vi "Acquire Data.vi"(4 "amplitude\nsweetspot":dbl, 6 "frequency\nsweetspot":dbl, 7 "error":bool, 10 "Amplitude":dbl, 11 "Frequency":dbl) -> (2 "FFTs":waveform(dbl)[](array[waveform]), 3 "Waveforms":waveform(dbl)[](array[waveform]))   [LabVIEW 2025, in "MCP Demo Application.lvlib"]
uses:
  MCP Demo Application.lvlib
  <vilib>/express/express analysis/Spectral/Block/exnSpectralBlock spectral measurements RMS poly.vi
  <vilib>/express/express analysis/Spectral/Block/exnSpectralBlock spectral measurements RMS array WFM.vi
  <vilib>/express/express analysis/Spectral/XNode/ExpressSpectralMeasurementsBlockNode.xnode
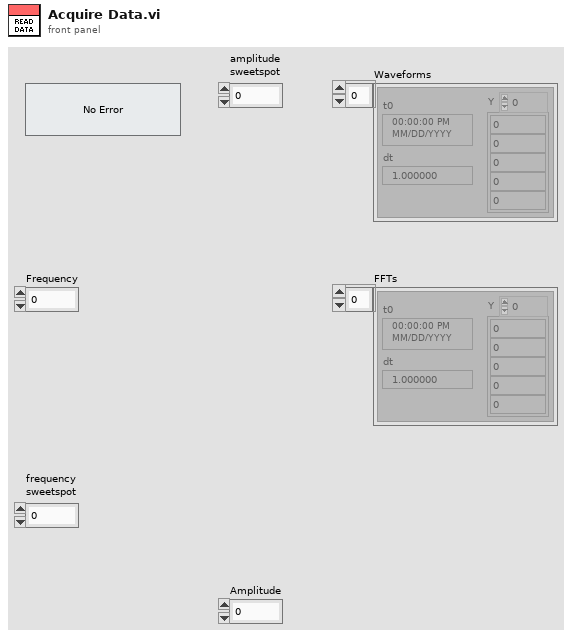
[diagram p1: front panel]
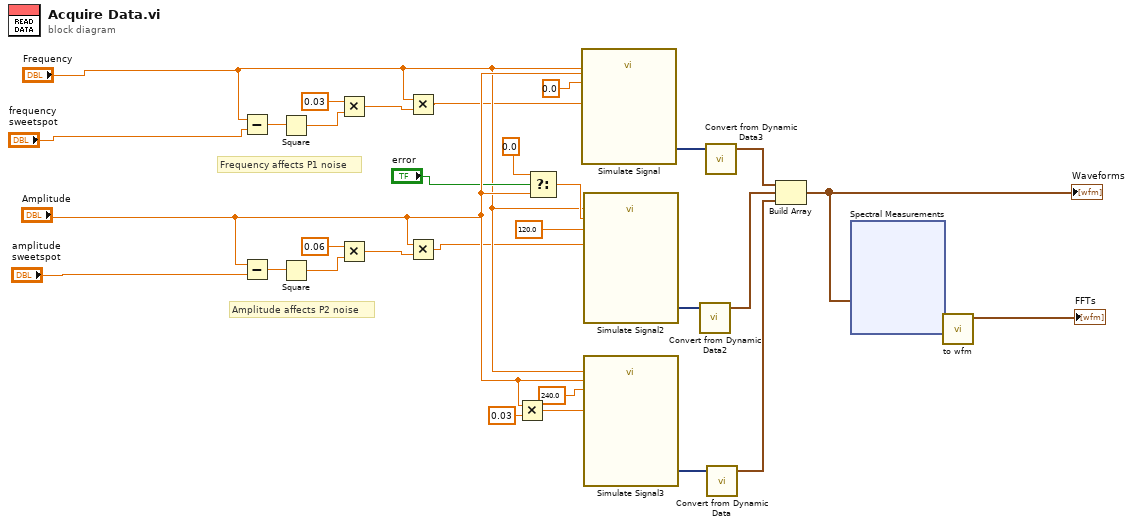
[diagram p0: block diagram]
diagram:
  # "Amplitude affects P2 noise"
  # "Frequency affects P1 noise"
  n1 = Subtract(x="Frequency", y="frequency\nsweetspot") -> (x-y=w20:dbl)
  n2 = Subtract(x="Amplitude", y="amplitude\nsweetspot") -> (x-y=w10:dbl)
  n3 = Square(x=w20) -> (x^2=w17:dbl)
  n4 = Square(x=w10) -> (x^2=w13:dbl)
  n5 = Multiply(x=0.03 ("Noise amplitude"), y=w17) -> (x*y=w18:dbl)
  n6 = Multiply(x=0.06 ("Noise amplitude"), y=w13) -> (x*y=w12:dbl)
  n7 = Multiply(x="Frequency", y=w18) -> (x*y=w21:dbl)
  n8 = Multiply(x="Amplitude", y=w12) -> (x*y=w14:dbl)
  n9 = Multiply(x="Amplitude", y=0.03) -> (x*y=w15:dbl)
  n10 = Select(t=0.0 ("Amplitude"), s="error", f="Amplitude") -> (s? t:f=w29:dbl)
  n11 = call "Simulate Signal"("Frequency"="Frequency", "Amplitude"="Amplitude", "Phase"=0.0, "Noise amplitude"=w21) -> ("P1"=w4:dynamicdata)  [unwired: 10 in, 1 out]
  n12 = call "Simulate Signal2"("Frequency"="Frequency", "Amplitude"=w29, "Phase"=120.0, "Noise amplitude"=w14) -> ("P2"=w5:dynamicdata)  [unwired: 10 in, 1 out]
  n13 = call "Simulate Signal3"("Frequency"="Frequency", "Amplitude"="Amplitude", "Phase"=240.0, "Noise amplitude"=w15) -> ("P3"=w6:dynamicdata)  [unwired: 10 in, 1 out]
  n14 = call "Convert from Dynamic Data2"("Dynamic Data Type"=w5) -> ("Waveform"=w8:waveform(dbl))  [unwired: 3 in]
  n15 = call "Convert from Dynamic Data3"("Dynamic Data Type"=w4) -> ("Waveform"=w7:waveform(dbl))  [unwired: 3 in]
  n16 = call "Convert from Dynamic Data"("Dynamic Data Type"=w6) -> ("Waveform"=w9:waveform(dbl))  [unwired: 3 in]
  n17 = Build Array(w7, w8, w9) -> (w27:waveform(dbl)[])
  "Waveforms" <- w27
  n18 = xnode "Spectral Measurements"("Signals"=w27) -> ("FFT - (RMS)"=w24:cluster{"f0":dbl, "df":dbl, "magnitude":dbl[]}[])  [unwired: 2 in, 3 out]
  n19 = call "to wfm.vi"("FFT - (RMS)"=w24) -> ("Array"=→"FFTs":waveform(dbl)[])  [unwired: 10 in]
